vi "FPGA VI_8 Channels_High Speed.vi"() -> ()   [LabVIEW 2015]
uses:
  FPGA/Injection Capture IP/Types/Injection.Timing.ctl
  FPGA/Injection Capture IP/Types/Injection.Core.Settings.ctl
  FPGA/Injection Capture IP/Types/Injection.Global.Settings.ctl
  <vilib>/rvi/eio/common/nirviEmuClasses.ctl
  FPGA/Injection Capture IP/Types/Injection.Mux.State.ctl
  <vilib>/Platform/TimedLoop/XDataNode/timing_clust.ctl
  <vilib>/Platform/TimedLoop/XDataNode/nitl_modes.ctl
  <vilib>/Platform/TimedLoop/XDataNode/wakeup.ctl
  FPGA/Injection Capture IP/Types/Injection.Core.Internal.Settings.ctl
  <vilib>/rvi/eio/common/nirviEmuTemplateMethod_errors.vi
  <vilib>/rvi/Emulation/niFpgaGetClockAttributes.vi
  <vilib>/rvi/Emulation/niFpgaSctlEmulationGetInTimedLoop.vi
  <vilib>/rvi/Emulation/niFpgaEmulationReportErrorSimple.vi
  <vilib>/rvi/Emulation/niFpgaCriticalErrorInLSC.vi
  <vilib>/rvi/eio/common/nirviEmuTemplateMethod_noerrors.vi
  <vilib>/rvi/DataTransferAndStorage/Container/Common/niFpgaContainerExecOnDevCompGetState.vi
  <vilib>/rvi/Emulation/niFpgaEmulationIsFPGAContextNoSignature.vi
  <vilib>/rvi/errors/niFpgaSetErrorForExecOnDevCompSimple.vi
  <vilib>/rvi/eio/common/nirviEmuReportErrorAndStop.vi
  <vilib>/rvi/DataTransferAndStorage/Container/Common/niFpgaContainerGetUniqueNameForEmu.vi
  <vilib>/rvi/FIFO/Fifo_Resource/nirvififoEmulationSetSize.vi
  <vilib>/rvi/FIFO/Fifo_Resource/nirviFifoEmulationQueueMgr.vi
  <instcachedir>/0/nirviFifoEmulationQueueMgr_E5CAEC123FF24DC58D834DCA3CDAA9B5.lvgen/nirviFifoEmulationQueueMgr_E5CAEC123FF24DC58D834DCA3CDAA9B5_010.vi
  <vilib>/rvi/FIFO/Fifo_Resource/nirvififoEmulationDetermineInputValidOut.vi
  <vilib>/rvi/FIFO/Fifo_Resource/nirvififoEmulationCreateLock.vi
  <vilib>/rvi/Emulation/niFpgaProcessEmulError.vi
  <vilib>/rvi/FIFO/Fifo_Resource/nirvififoEmulationObtainLock.vi
  <vilib>/rvi/FIFO/Fifo_Resource/nirvififoEmulationReleaseLock.vi
  <vilib>/rvi/occurrence/nirviWaitOnOccurrenceBase.vi
  <vilib>/rvi/errors/nirviReportUnexpectedCaseInternalError.vi
  <vilib>/rvi/errors/nirviReportUnexpectedCaseInternalError (U32).vi
  <vilib>/Utility/error.llb/Clear Errors.vi
  <vilib>/rvi/interface/RandomDataEmulation/niFpgaRandomDataHandleErrors.vi
  <instcachedir>/0/nirviFifoEmulationQueueMgr_E5CAEC123FF24DC58D834DCA3CDAA9B5.lvgen/nirviFifoEmulationQueueMgr_E5CAEC123FF24DC58D834DCA3CDAA9B5_008.vi
  <vilib>/eio/EIOGrowableMethodNode/genericMethod/EIOGrowableMethodNode.xnode
  <vilib>/rvi/eio/nirviEIOMethodImplementation/nirviEIOMethodImplementation.xnode
  <vilib>/rvi/eio/nirviErrorMerge/nirviErrorMerge.xnode
  <vilib>/Platform/TimedLoop/XDataNode/XDataNode.xnode
  <vilib>/rvi/DataTransferAndStorage/Container/XNode/niFpgaContainer.xnode
  <vilib>/rvi/FIFO/Fifo_Resource/niFpgaFifoEmulationRefIn.vi
  <vilib>/rvi/interface/RandomDataEmulation/nirviRandomDataFpgaReadWriteTemplate.vi
  <vilib>/Platform/TimedLoop/XDataNode/XDNodeRunTimeDep.lvlib
panel:
  in  "Settings.DMA":cluster{"# of Injectors":u8}={"# of Injectors"=6}
  out "Host DMA Out?":bool
  out "Intermediate Time Out?":bool
  out "Sample Clock Ticks":u32
  out "Module Error":bool
  out "Module Initialization Error Code":i32
  out "IO Node Timeout":bool
  in  "Settings.Index6.Injectors.Injector6":T1
  in  "Settings.Index7.Injectors.Injector7":T1
  out "Intermediate FIFO Write Timeout":bool
  in  "Settings.Global.Injectors":T2={"Enable?"=FALSE, "Initial Voltage Threshold"=12.0, "Event Dwell Limit"=2000, "Voltage Gain"=1.0, "Current Gain"=1.0, "Filter Samples"=5, "Pretrigger Samples"=5}
  in  "Settings.Index0.Injectors.Injector0":T1
  in  "Settings.Index1.Injectors.Injector1":T1
  in  "Settings.Index2.Injectors.Injector2":T1
  in  "Settings.Index3.Injectors.Injector3":T1
  in  "Settings.Index4.Injectors.Injector4":T1
  in  "Settings.Index5.Injectors.Injector5":T1
  in  "Settings.Timing":T3={"Injection Sample Period (Ticks)"=80}
  out "Acqusition Loop Ticks":u32
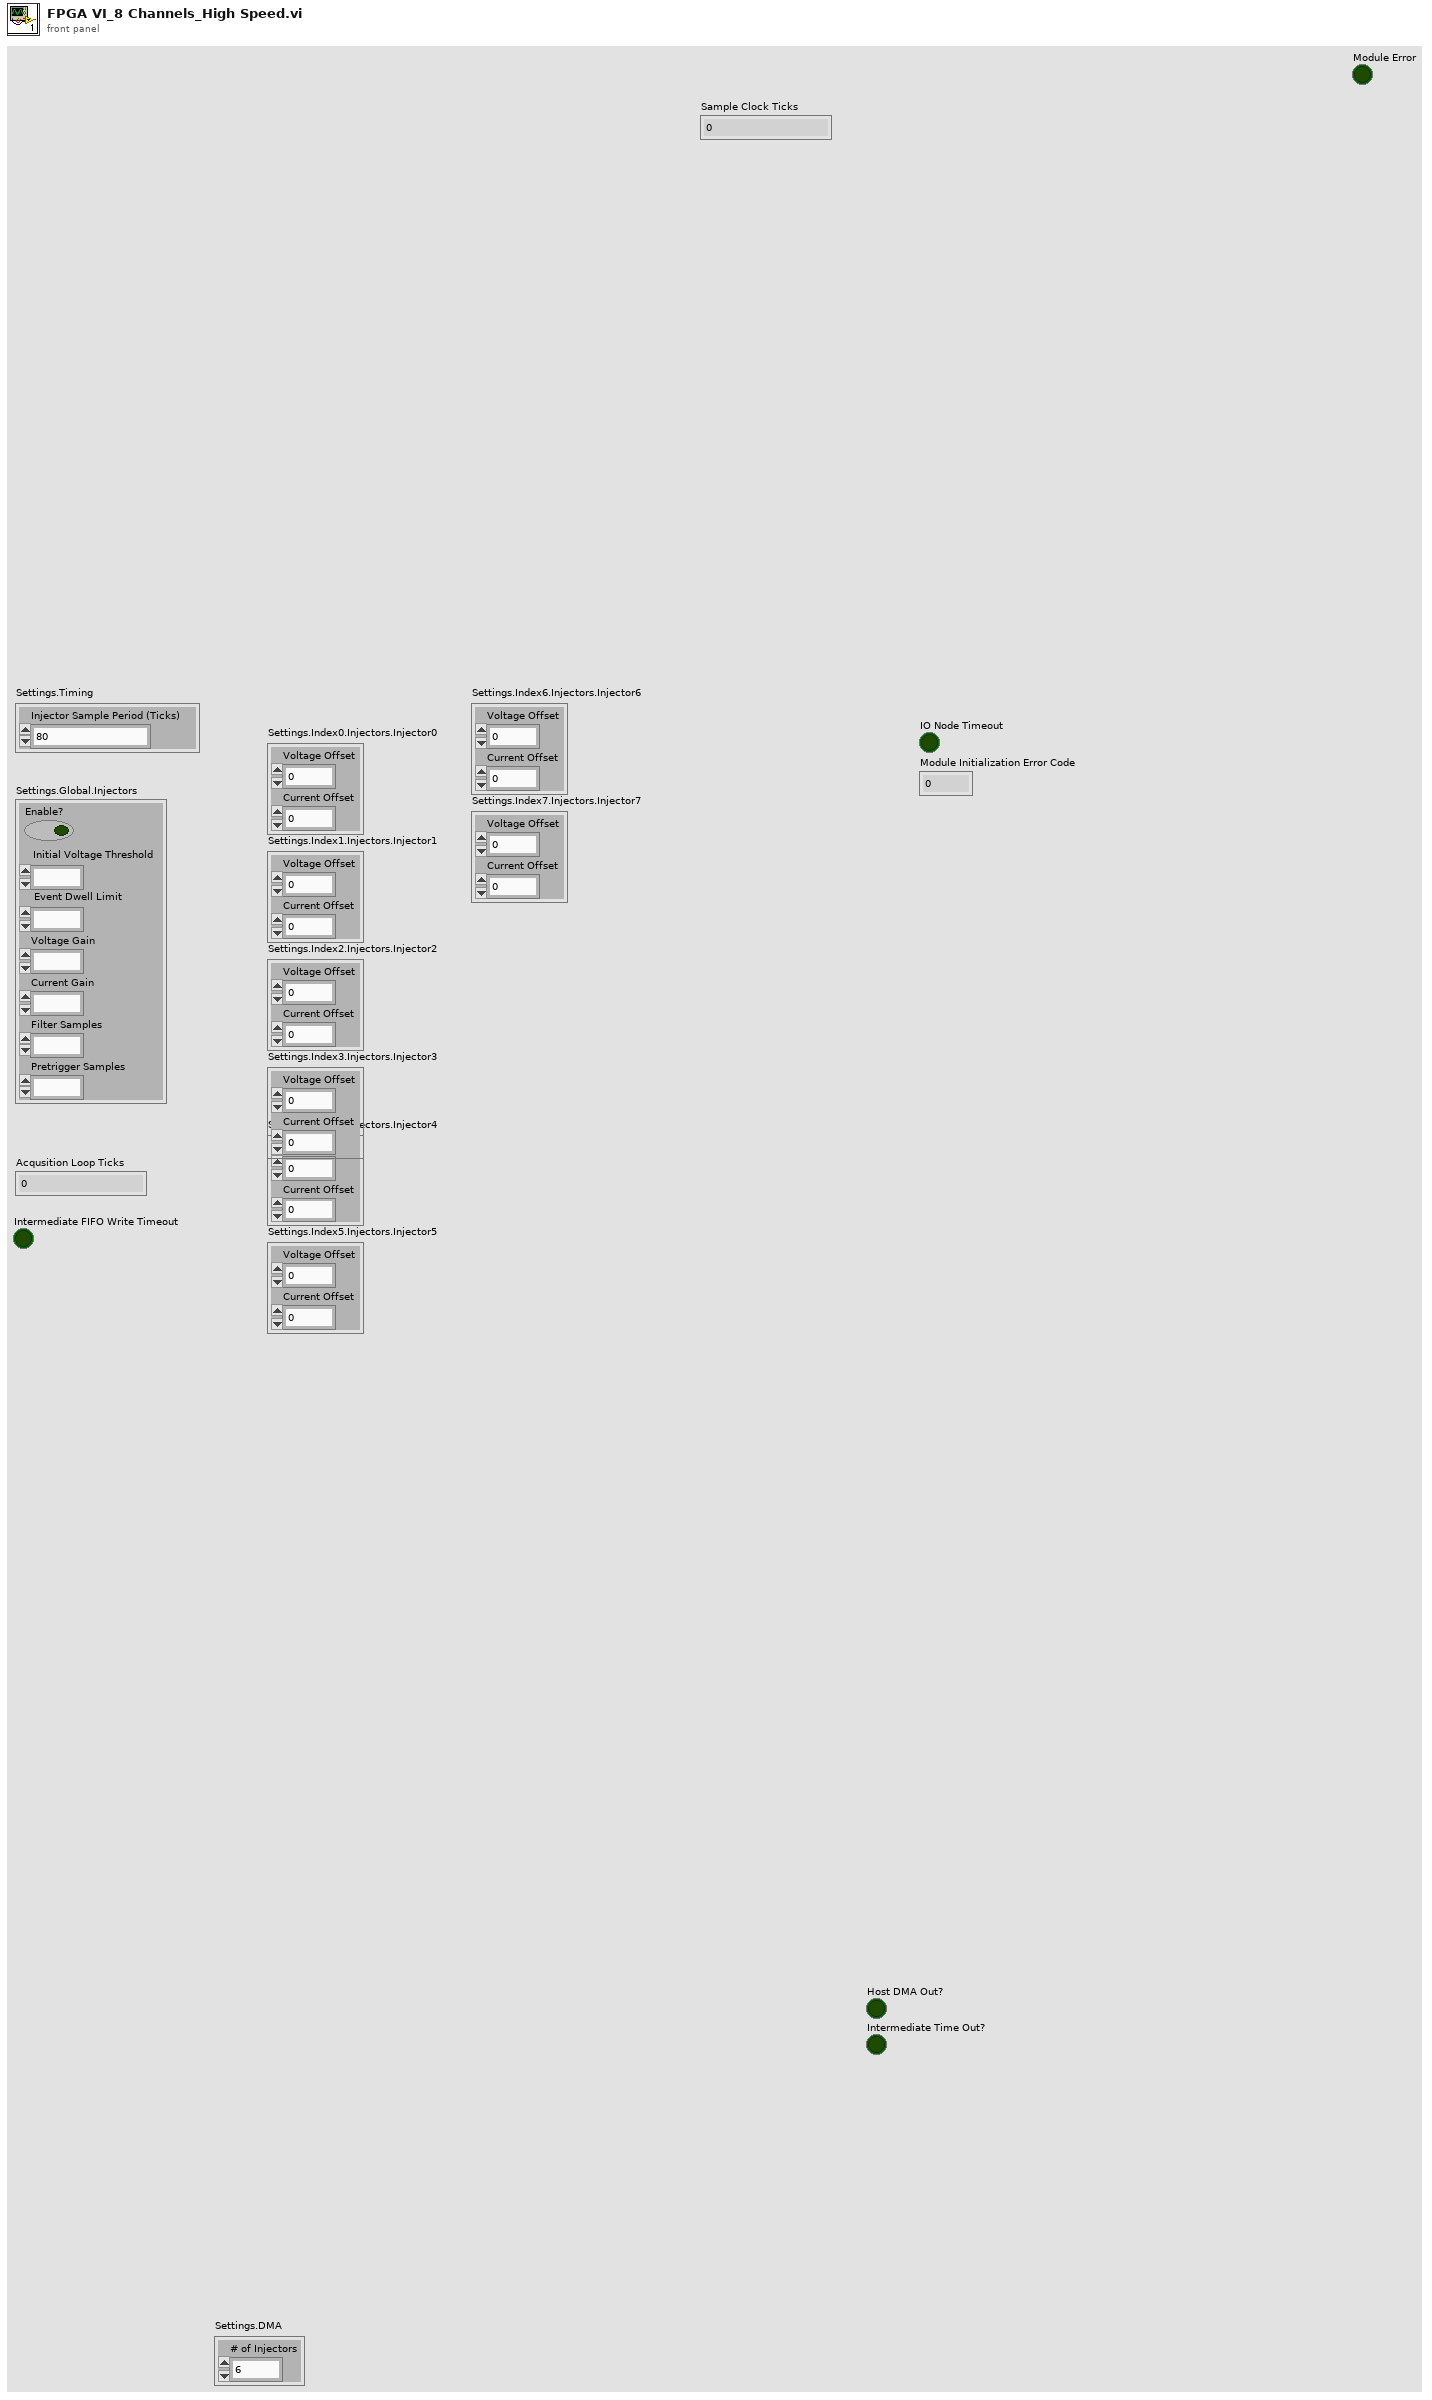
[diagram p1: front panel]
types:
  T1 = typedef "Injection.Core.Settings.ctl" = cluster{"Voltage Offset":fxp<+/-,32,8>, "Current Offset":fxp<+/-,32,8>}
  T2 = typedef "Injection.Global.Settings.ctl" = cluster{"Enable?":bool, "Initial Voltage Threshold":fxp<+/-,32,8>, "Event Dwell Limit":u16, "Voltage Gain":fxp<+/-,32,8>, "Current Gain":fxp<+/-,32,8>, "Filter Samples":u8, "Pretrigger Samples":u8}
  T3 = typedef "Injection.Timing.ctl" = cluster{"Injection Sample Period (Ticks)":u32}
  T4 = typedef "nirviEmuClasses.ctl" = enum16{"IO Read", "IO Write", "Method", "Property Read", "Property Write"}
  T5 = cluster{"Data.Samples":u32, "Injection.Period":u32, "Injector.Index":u8, "Iteration":u32}
  T6 = typedef "Injection.Mux.State.ctl" = enum8{"Wait on Transfer", "Transfer Injector Index", "Transfer # of Samples", "Transfer Injection Period", "Transfer Data Samples"}
  T7 = typedef "XDNodeRunTimeDep.lvlib/timing_clust.ctl" = cluster{"Expected End [f-1]":u64, "Actual End [f-1]":u64, "Finished Late? [f-1]":bool, "Expected End [i-1]":u64, "Actual End [i-1]":u64, "Finished Late? [i-1]":bool, "Expected Start [i]":u64, "Actual Start [i]":u64, "Expected Start [f]":u64, "Actual Start [f]":u64, "Source Name":string, "Structure Name":string, "Period":i64, "Deadline":i64, "Offset":i64, "Start":i64, "Priority":i32, "Timeout":i32, "Mode":T8, "Wakeup Reason":T9, "Error":errorcluster, "Source Type":string, "Secondary Source Type":string, "Global End Time":u64, "Global Start Time":u64, "Frame Duration":u64, "Iteration Duration":u64, "Assigned CPU":i32, "I/O Scan Engine Mode":u32}
  T8 = typedef "XDNodeRunTimeDep.lvlib/nitl_modes.ctl" = enum32{"No Change", "Process missed periods, maintain original phase", "Discard missed periods, maintain original phase", "Process missed periods, ignore original phase", "Discard missed periods, ignore original phase"}
  T9 = typedef "XDNodeRunTimeDep.lvlib/wakeup.ctl" = enum32{"Normal", "Aborted", "Asynchronous wakeup", "Timing source error", "Timed loop error", "Timeout"}
  T10 = typedef "Injection.Core.Internal.Settings.ctl" = cluster{"Data Buffer FIFO":refnum<k21>, "Capture Complete Trigger FIFO":refnum<k21>}
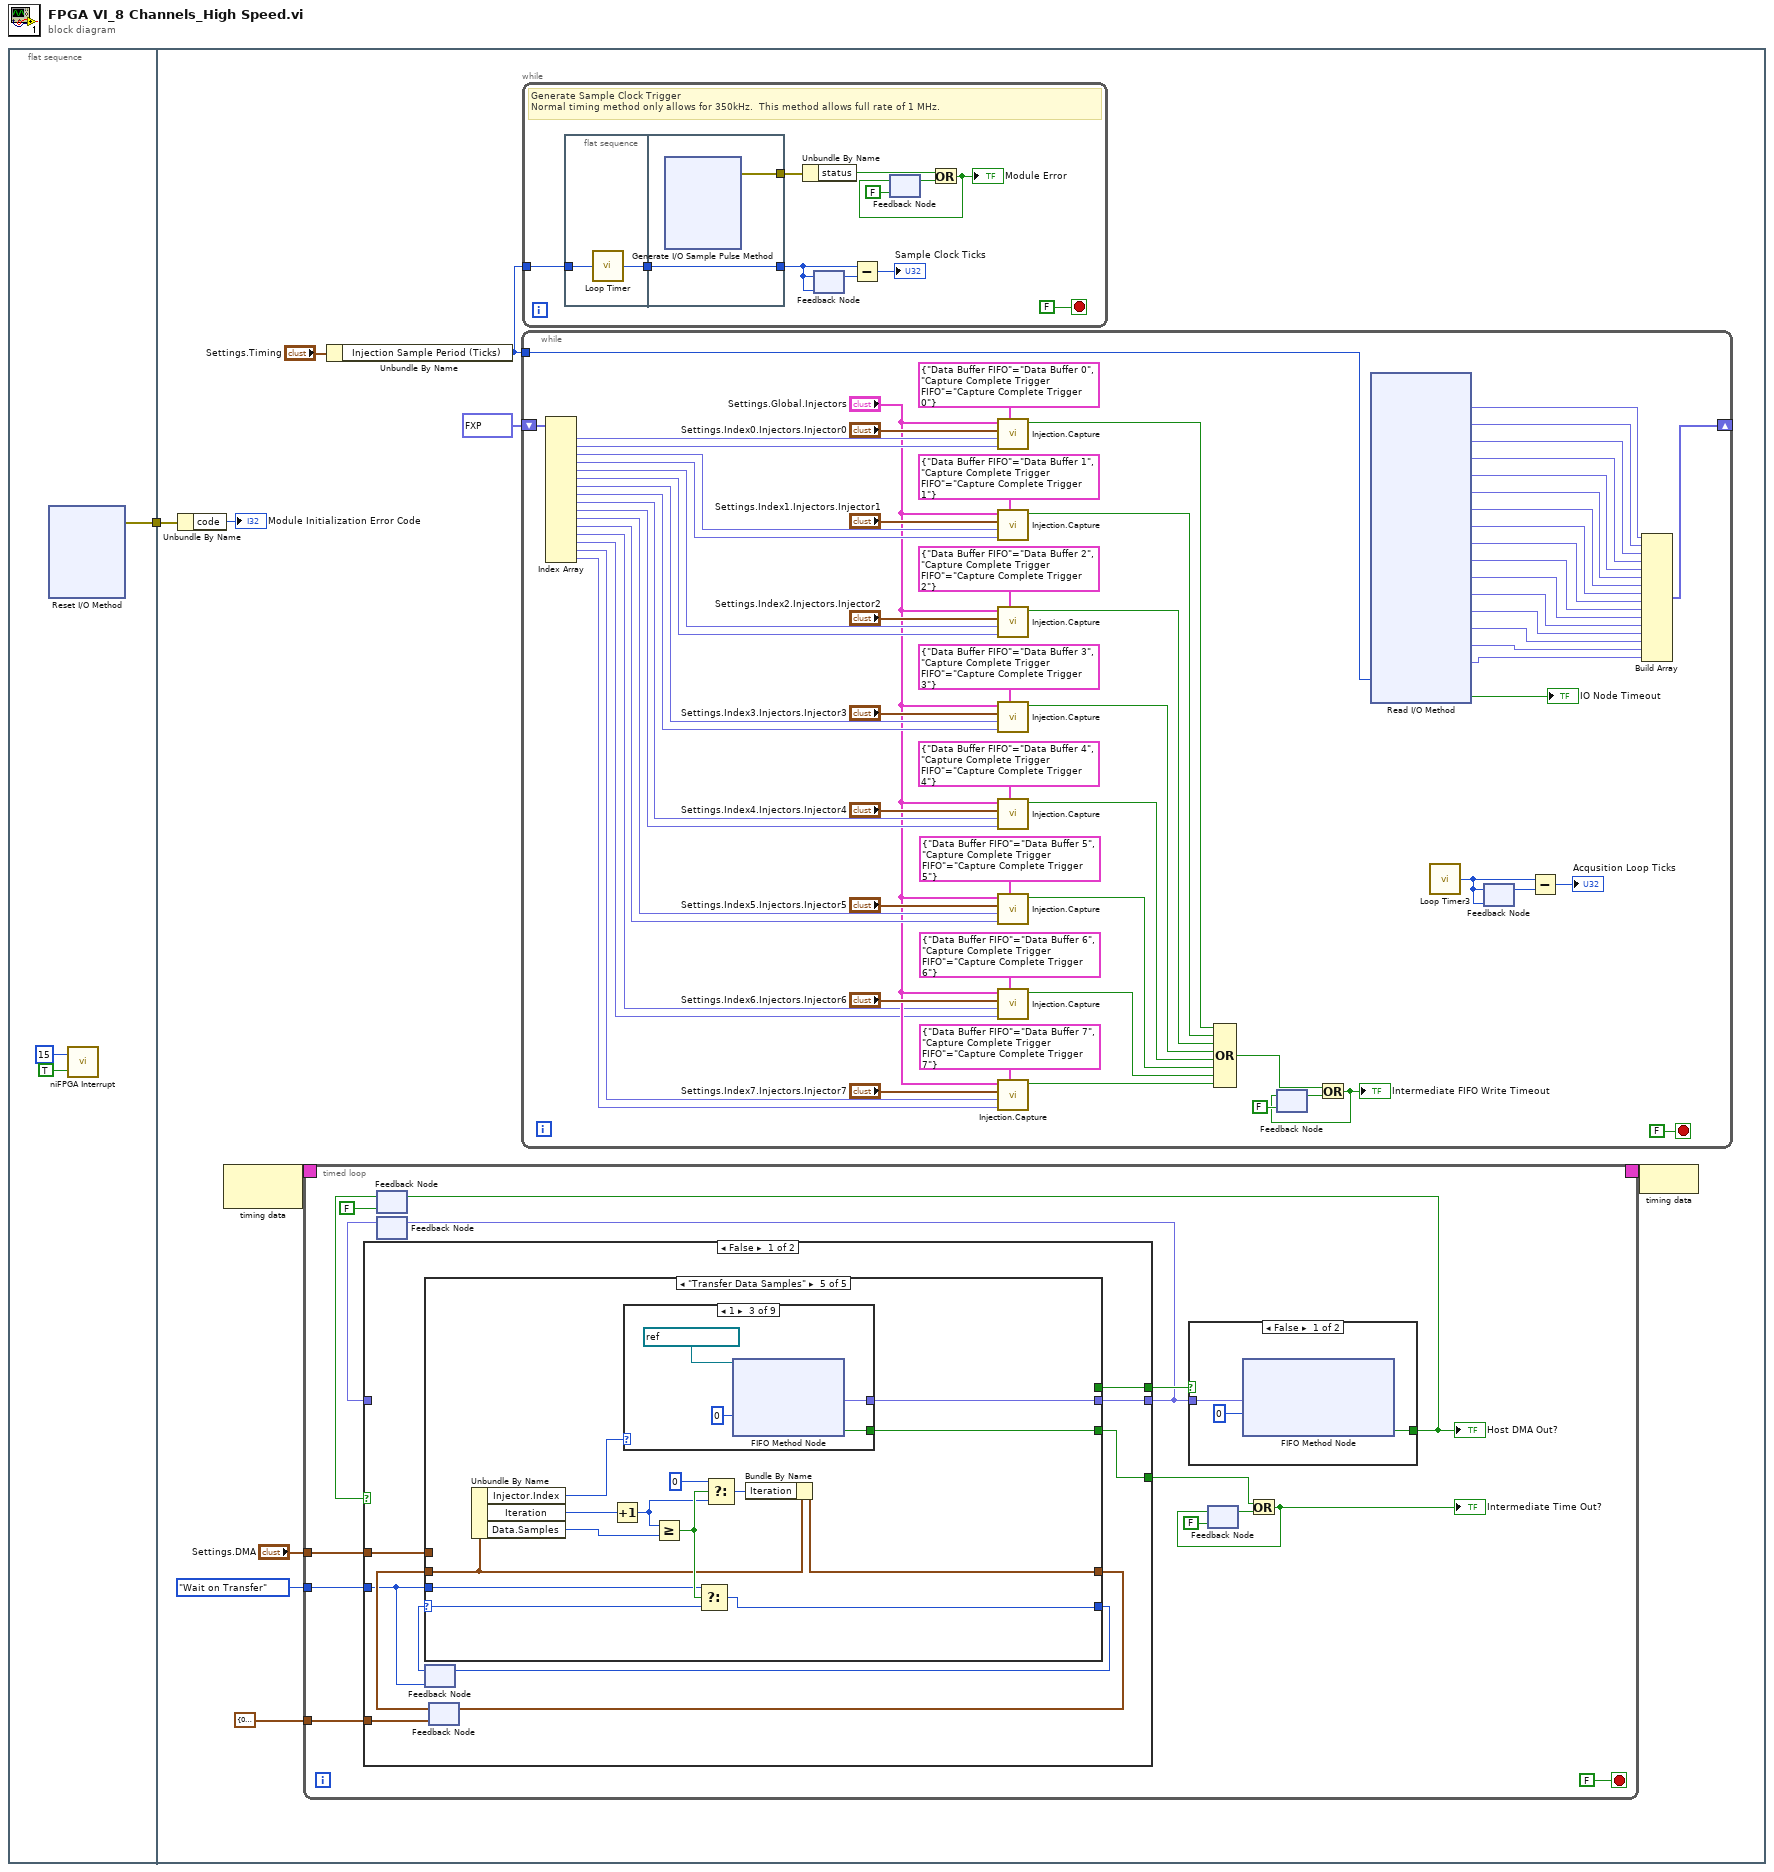
[diagram p0: block diagram]
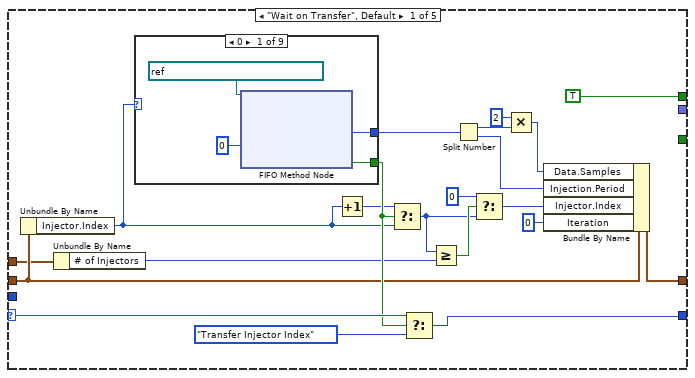
[diagram p2: hidden frame]
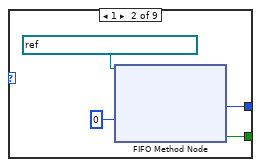
[diagram p3: hidden frame]
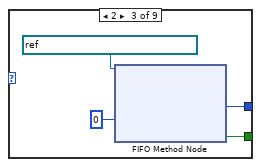
[diagram p4: hidden frame]
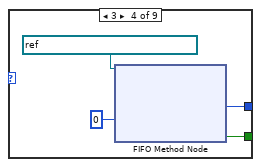
[diagram p5: hidden frame]
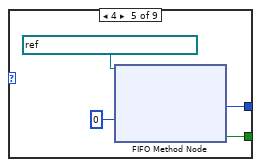
[diagram p6: hidden frame]
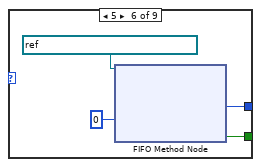
[diagram p7: hidden frame]
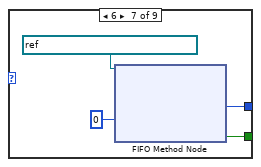
[diagram p8: hidden frame]
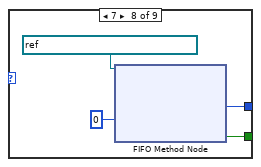
[diagram p9: hidden frame]
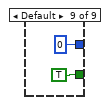
[diagram p10: hidden frame]
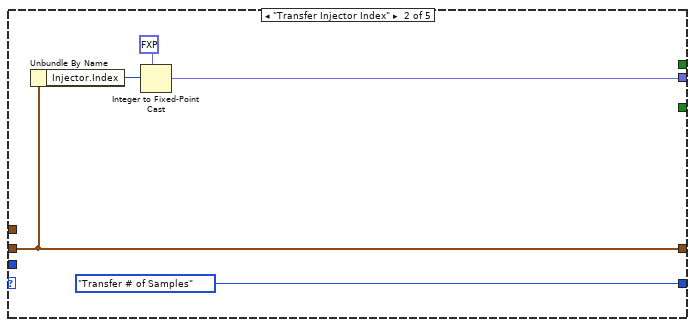
[diagram p11: hidden frame]
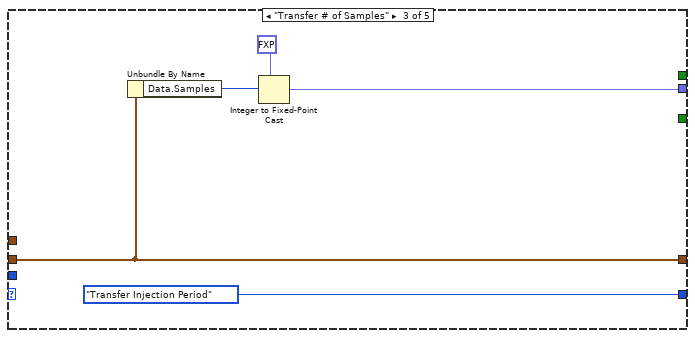
[diagram p12: hidden frame]
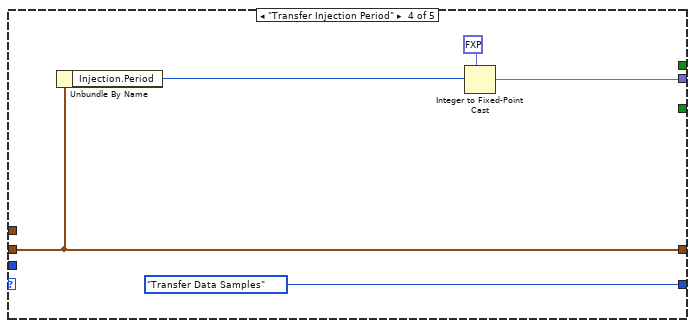
[diagram p13: hidden frame]
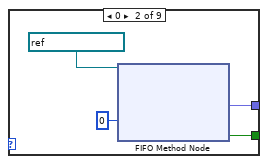
[diagram p15: hidden frame]
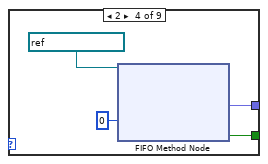
[diagram p16: hidden frame]
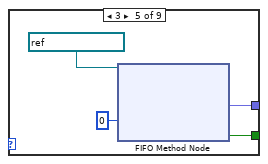
[diagram p17: hidden frame]
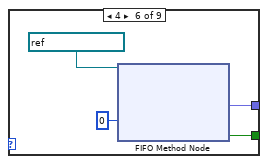
[diagram p18: hidden frame]
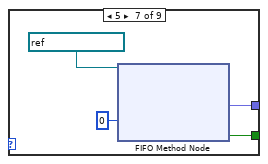
[diagram p19: hidden frame]
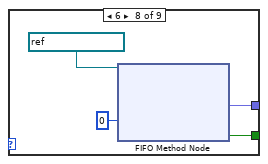
[diagram p20: hidden frame]
diagram:
  n1 = flat-sequence {
    tunnel: [w2] -> w1
    tunnel: w1 -> [w86]
    frame #0 {
      n2 = xnode "Reset I/O Method"() -> ("error out"=w2:errorcluster)  [unwired: 5 in, 4 out]
      n3 = call <vilib>:"niFPGA Interrupt.vi"("Wait Until Cleared (F)"=TRUE, "IRQ Number (0)"=u8 15) -> ()  [unwired: 1 in]
    }
    frame #1 {
      n4 = Unbundle By Name(w86) -> ("code"=→"Module Initialization Error Code":i32)
      n5 = node-c288() -> (w83:T7)  [unwired: 1 in]
      n6 = timed-loop {
        timing: w83 -> [_]
        timing-out: [_] -> w82
        tunnel: "Settings.DMA" -> [w92]
        tunnel: Injection.Mux.State."Wait on Transfer" -> [w91]
        tunnel: T5 {"Data.Samples"=0, "Injection.Period"=0, "Injector.Index"=0, "Iteration"=0} ("Local.Data") -> [w90]
        stop <- FALSE stop-if-true
        n7 = feedback #1(FALSE ("Timed Out?")) -> (w100:bool)
        n8 = feedback #2() -> (w97:fxp<+/-,32,8>)  [unwired: 1 in]
        n9 = case shown="False" w100 {
          tunnel: [w112 w230] -> w98
          tunnel: [w111 w229] -> w102
          tunnel: w91 -> [w105 _]
          tunnel: [w110 w229] -> w93
          tunnel: w92 -> [w109 _]
          tunnel: w90 -> [w106 _]
          tunnel: w97 -> [_ w230]
          frame False {
            n10 = feedback #3(w105) -> (w104:T6)
            n11 = feedback #4(w106) -> (w107:T5)
            n12 = case shown="\"Transfer Data Samples\"" w104 {
              selector: w104 -> [w133 _ _ _ w190]
              tunnel: w107 -> [w124 w171 w175 w179 w188]
              tunnel: [w132 w171 w175 w179 w187] -> w108
              tunnel: [w131 Injection.Mux.State."Transfer # of Samples" Injection.Mux.State."Transfer Injection Period" Injection.Mux.State."Transfer Data Samples" w189] -> w103
              tunnel: [_ w170 w174 w181 w186] -> w112
              tunnel: [TRUE _ _ _ _] -> w111
              tunnel: w105 -> [_ _ _ _ w183]
              tunnel: [_ _ _ _ w185] -> w110
              tunnel: w109 -> [w121 _ _ _ _]
              frame "Wait on Transfer", Default {
                n13 = Unbundle By Name(w124) -> ("Injector.Index"=w123:u8)
                n14 = Unbundle By Name(w121) -> ("# of Injectors"=w120:u8)
                n15 = case shown="0" w123 {
                  tunnel: [w136 w140 w144 w148 w152 w156 w160 w164 u64 0 ("Element")] -> w119
                  tunnel: [w135 w139 w143 w147 w151 w155 w159 w163 TRUE ("Timed Out?")] -> w129
                  frame 0 {
                    n16 = xnode ("FIFO Method Node")("Timeout"=0, "FIFO In"=refnum<k21> "Capture Complete Trigger 0") -> ("Element"=w136:u64, "Timed Out?"=w135:bool)  [unwired: 1 out]
                  }
                  frame 1 {
                    n17 = xnode ("FIFO Method Node")("Timeout"=0, "FIFO In"=refnum<k21> "Capture Complete Trigger 1") -> ("Element"=w140:u64, "Timed Out?"=w139:bool)  [unwired: 1 out]
                  }
                  frame 2 {
                    n18 = xnode ("FIFO Method Node")("Timeout"=0, "FIFO In"=refnum<k21> "Capture Complete Trigger 2") -> ("Element"=w144:u64, "Timed Out?"=w143:bool)  [unwired: 1 out]
                  }
                  frame 3 {
                    n19 = xnode ("FIFO Method Node")("Timeout"=0, "FIFO In"=refnum<k21> "Capture Complete Trigger 3") -> ("Element"=w148:u64, "Timed Out?"=w147:bool)  [unwired: 1 out]
                  }
                  frame 4 {
                    n20 = xnode ("FIFO Method Node")("Timeout"=0, "FIFO In"=refnum<k21> "Capture Complete Trigger 4") -> ("Element"=w152:u64, "Timed Out?"=w151:bool)  [unwired: 1 out]
                  }
                  frame 5 {
                    n21 = xnode ("FIFO Method Node")("Timeout"=0, "FIFO In"=refnum<k21> "Capture Complete Trigger 5") -> ("Element"=w156:u64, "Timed Out?"=w155:bool)  [unwired: 1 out]
                  }
                  frame 6 {
                    n22 = xnode ("FIFO Method Node")("Timeout"=0, "FIFO In"=refnum<k21> "Capture Complete Trigger 6") -> ("Element"=w160:u64, "Timed Out?"=w159:bool)  [unwired: 1 out]
                  }
                  frame 7 {
                    n23 = xnode ("FIFO Method Node")("Timeout"=0, "FIFO In"=refnum<k21> "Capture Complete Trigger 7") -> ("Element"=w164:u64, "Timed Out?"=w163:bool)  [unwired: 1 out]
                  }
                  frame Default {
                  }
                }
                n24 = Increment(x=w123) -> (x+1=w128:u8)
                n25 = Select(t=w128, s=w129, f=w123) -> (s? t:f=w126:u8)
                n26 = Select(t=w133, s=w129, f=Injection.Mux.State."Transfer Injector Index") -> (s? t:f=w131:T6)
                n27 = Greater Or Equal?(x=w126, y=w120) -> (x >= y?=w127:bool)
                n28 = Split Number(x=w119) -> (hi(x)=w118:u32, lo(x)=w117:u32)
                n29 = Select(t=u8 0, s=w127, f=w126) -> (s? t:f=w122:u8)
                n30 = Multiply(x=u32 2, y=w118) -> (x*y=w115:u32)
                n31 = Bundle By Name(cluster=w124, "Data.Samples"=w115, "Injection.Period"=w117, "Injector.Index"=w122, "Iteration"=u32 0) -> (w132:T5)
              }
              frame "Transfer Injector Index" {
                n32 = Unbundle By Name(w171) -> ("Injector.Index"=w172:u8)
                n33 = Integer to Fixed-Point Cast(fixed-point type=fxp<+/-,32,8> 0.0, integer=w172) -> (fixed-point=w170:fxp<+/-,32,8>)
              }
              frame "Transfer # of Samples" {
                n34 = Unbundle By Name(w175) -> ("Data.Samples"=w176:u32)
                n35 = Integer to Fixed-Point Cast(fixed-point type=fxp<+/-,32,8> 0.0, integer=w176) -> (fixed-point=w174:fxp<+/-,32,8>)
              }
              frame "Transfer Injection Period" {
                n36 = Unbundle By Name(w179) -> ("Injection.Period"=w180:u32)
                n37 = Integer to Fixed-Point Cast(fixed-point type=fxp<+/-,32,8> 0.0, integer=w180) -> (fixed-point=w181:fxp<+/-,32,8>)
              }
              frame "Transfer Data Samples" {
                n38 = Unbundle By Name(w188) -> ("Injector.Index"=w196:u8, "Iteration"=w191:u32, "Data.Samples"=w184:u32)
                n39 = Increment(x=w191) -> (x+1=w193:u32)
                n40 = case shown="1" w196 {
                  tunnel: [_ w199 w203 w207 w211 w215 w219 w223 w227] -> w186
                  tunnel: [_ w198 w202 w206 w210 w214 w218 w222 w226] -> w185
                  frame Default {
                  }
                  frame 0 {
                    n41 = xnode ("FIFO Method Node")("Timeout"=0, "FIFO In"=refnum<k21> "Data Buffer 0" ("Voltage FIFO")) -> ("Element"=w199:fxp<+/-,32,8>, "Timed Out?"=w198:bool)  [unwired: 1 out]
                  }
                  frame 1 {
                    n42 = xnode ("FIFO Method Node")("Timeout"=0, "FIFO In"=refnum<k21> "Data Buffer 1" ("Voltage FIFO")) -> ("Element"=w203:fxp<+/-,32,8>, "Timed Out?"=w202:bool)  [unwired: 1 out]
                  }
                  frame 2 {
                    n43 = xnode ("FIFO Method Node")("Timeout"=0, "FIFO In"=refnum<k21> "Data Buffer 2" ("Voltage FIFO")) -> ("Element"=w207:fxp<+/-,32,8>, "Timed Out?"=w206:bool)  [unwired: 1 out]
                  }
                  frame 3 {
                    n44 = xnode ("FIFO Method Node")("Timeout"=0, "FIFO In"=refnum<k21> "Data Buffer 3" ("Voltage FIFO")) -> ("Element"=w211:fxp<+/-,32,8>, "Timed Out?"=w210:bool)  [unwired: 1 out]
                  }
                  frame 4 {
                    n45 = xnode ("FIFO Method Node")("Timeout"=0, "FIFO In"=refnum<k21> "Data Buffer 4" ("Voltage FIFO")) -> ("Element"=w215:fxp<+/-,32,8>, "Timed Out?"=w214:bool)  [unwired: 1 out]
                  }
                  frame 5 {
                    n46 = xnode ("FIFO Method Node")("Timeout"=0, "FIFO In"=refnum<k21> "Data Buffer 5" ("Voltage FIFO")) -> ("Element"=w219:fxp<+/-,32,8>, "Timed Out?"=w218:bool)  [unwired: 1 out]
                  }
                  frame 6 {
                    n47 = xnode ("FIFO Method Node")("Timeout"=0, "FIFO In"=refnum<k21> "Data Buffer 6" ("Voltage FIFO")) -> ("Element"=w223:fxp<+/-,32,8>, "Timed Out?"=w222:bool)  [unwired: 1 out]
                  }
                  frame 7 {
                    n48 = xnode ("FIFO Method Node")("Timeout"=0, "FIFO In"=refnum<k21> "Data Buffer 7" ("Voltage FIFO")) -> ("Element"=w227:fxp<+/-,32,8>, "Timed Out?"=w226:bool)  [unwired: 1 out]
                  }
                }
                n49 = Greater Or Equal?(x=w193, y=w184) -> (x >= y?=w195:bool)
                n50 = Select(t=w183, s=w195, f=w190) -> (s? t:f=w189:T6)
                n51 = Select(t=u32 0, s=w195, f=w193) -> (s? t:f=w192:u32)
                n52 = Bundle By Name(cluster=w188, "Iteration"=w192) -> (w187:T5)
              }
            }
            n53 = feedback-in #3(w103) -> ()
            n54 = feedback-in #4(w108) -> ()
          }
          frame True {
            w229 = FALSE
          }
        }
        n55 = feedback-in #2(w98) -> ()
        n56 = case shown="False" w102 {
          tunnel: w98 -> [w232 _]
          tunnel: [w231 FALSE ("Timed Out?")] -> w101
          frame False {
            n57 = xnode ("FIFO Method Node")("Element"=w232, "Timeout"=0) -> ("Timed Out?"=w231:bool)  [unwired: 1 in, 1 out]
          }
          frame True {
          }
        }
        "Host DMA Out?" <- w101
        n58 = feedback-in #1(w101) -> ()
        n59 = feedback #5(FALSE ("Timed Out?")) -> (w95:bool)
        n60 = Or(x=w93, y=w95) -> (x .or. y?=w94:bool)
        "Intermediate Time Out?" <- w94
        n61 = feedback-in #5(w94) -> ()
      }
      n62 = Unbundle By Name("Settings.Timing") -> ("Injection Sample Period (Ticks)"=w84:u32)
      n63 = while {
        shift-right: [w268] -> _
        shift-left: fxp<+/-,24,5>[] [0.0, 0.0, 0.0, 0.0, 0.0, 0.0, 0.0, 0.0, 0.0, 0.0, 0.0, 0.0, 0.0, 0.0, 0.0, 0.0] -> [w288]
        tunnel: w84 -> [w239]
        stop <- FALSE stop-if-true
        n64 = Index Array(array=w288) -> (element #1=w299:fxp<+/-,24,5>, element #2=w300:fxp<+/-,24,5>, element #3=w297:fxp<+/-,24,5>, element #4=w298:fxp<+/-,24,5>, element #5=w295:fxp<+/-,24,5>, element #6=w296:fxp<+/-,24,5>, element #7=w293:fxp<+/-,24,5>, element #8=w294:fxp<+/-,24,5>, element #9=w291:fxp<+/-,24,5>, element #10=w292:fxp<+/-,24,5>, element #11=w289:fxp<+/-,24,5>, element #12=w290:fxp<+/-,24,5>, element #13=w260:fxp<+/-,24,5>, element #14=w259:fxp<+/-,24,5>, element #15=w258:fxp<+/-,24,5>, element #16=w257:fxp<+/-,24,5>)  [unwired: 16 in]
        n65 = call "Injection.Capture.vi"("FIFOs"=T10 {"Data Buffer FIFO"="Data Buffer 0", "Capture Complete Trigger FIFO"="Capture Complete Trigger 0"} ("InjectorCore.Settings"), "Current (PreScaled)"=w300, "Voltage (PreScaled)"=w299, "Settings.Index<#>.<Group>.<UserName>"="Settings.Index0.Injectors.Injector0", "Settings.Global.<Group>"="Settings.Global.Injectors") -> ("Intermediate FIFO Timeout?"=w307:bool)  [unwired: 4 in, 2 out]
        n66 = call "Injection.Capture.vi"("FIFOs"=T10 {"Data Buffer FIFO"="Data Buffer 1", "Capture Complete Trigger FIFO"="Capture Complete Trigger 1"} ("InjectorCore.Settings"), "Current (PreScaled)"=w298, "Voltage (PreScaled)"=w297, "Settings.Index<#>.<Group>.<UserName>"="Settings.Index1.Injectors.Injector1", "Settings.Global.<Group>"="Settings.Global.Injectors") -> ("Intermediate FIFO Timeout?"=w306:bool)  [unwired: 4 in, 2 out]
        n67 = call "Injection.Capture.vi"("FIFOs"=T10 {"Data Buffer FIFO"="Data Buffer 2", "Capture Complete Trigger FIFO"="Capture Complete Trigger 2"} ("InjectorCore.Settings"), "Current (PreScaled)"=w296, "Voltage (PreScaled)"=w295, "Settings.Index<#>.<Group>.<UserName>"="Settings.Index2.Injectors.Injector2", "Settings.Global.<Group>"="Settings.Global.Injectors") -> ("Intermediate FIFO Timeout?"=w305:bool)  [unwired: 4 in, 2 out]
        n68 = call "Injection.Capture.vi"("FIFOs"=T10 {"Data Buffer FIFO"="Data Buffer 3", "Capture Complete Trigger FIFO"="Capture Complete Trigger 3"} ("InjectorCore.Settings"), "Current (PreScaled)"=w294, "Voltage (PreScaled)"=w293, "Settings.Index<#>.<Group>.<UserName>"="Settings.Index3.Injectors.Injector3", "Settings.Global.<Group>"="Settings.Global.Injectors") -> ("Intermediate FIFO Timeout?"=w304:bool)  [unwired: 4 in, 2 out]
        n69 = call "Injection.Capture.vi"("FIFOs"=T10 {"Data Buffer FIFO"="Data Buffer 4", "Capture Complete Trigger FIFO"="Capture Complete Trigger 4"} ("InjectorCore.Settings"), "Current (PreScaled)"=w292, "Voltage (PreScaled)"=w291, "Settings.Index<#>.<Group>.<UserName>"="Settings.Index4.Injectors.Injector4", "Settings.Global.<Group>"="Settings.Global.Injectors") -> ("Intermediate FIFO Timeout?"=w303:bool)  [unwired: 4 in, 2 out]
        n70 = call "Injection.Capture.vi"("FIFOs"=T10 {"Data Buffer FIFO"="Data Buffer 5", "Capture Complete Trigger FIFO"="Capture Complete Trigger 5"} ("InjectorCore.Settings"), "Current (PreScaled)"=w290, "Voltage (PreScaled)"=w289, "Settings.Index<#>.<Group>.<UserName>"="Settings.Index5.Injectors.Injector5", "Settings.Global.<Group>"="Settings.Global.Injectors") -> ("Intermediate FIFO Timeout?"=w302:bool)  [unwired: 4 in, 2 out]
        n71 = call "Injection.Capture.vi"("FIFOs"=T10 {"Data Buffer FIFO"="Data Buffer 6", "Capture Complete Trigger FIFO"="Capture Complete Trigger 6"} ("InjectorCore.Settings"), "Current (PreScaled)"=w259, "Voltage (PreScaled)"=w260, "Settings.Index<#>.<Group>.<UserName>"="Settings.Index6.Injectors.Injector6", "Settings.Global.<Group>"="Settings.Global.Injectors") -> ("Intermediate FIFO Timeout?"=w262:bool)  [unwired: 4 in, 2 out]
        n72 = call "Injection.Capture.vi"("FIFOs"=T10 {"Data Buffer FIFO"="Data Buffer 7", "Capture Complete Trigger FIFO"="Capture Complete Trigger 7"} ("InjectorCore.Settings"), "Current (PreScaled)"=w257, "Voltage (PreScaled)"=w258, "Settings.Index<#>.<Group>.<UserName>"="Settings.Index7.Injectors.Injector7", "Settings.Global.<Group>"="Settings.Global.Injectors") -> ("Intermediate FIFO Timeout?"=w261:bool)  [unwired: 4 in, 2 out]
        n73 = Compound Arithmetic op=OR(w307, w306, w305, w304, w303, w302, w262, w261) -> (w278:bool)
        n74 = feedback #6(FALSE ("Timed Out?")) -> (w279:bool)
        n75 = Or(x=w278, y=w279) -> (x .or. y?=w277:bool)
        "Intermediate FIFO Write Timeout" <- w277
        n76 = feedback-in #6(w277) -> ()
        n77 = xnode "Read I/O Method"("Timeout"=w239) -> ("Mod1/AI0"=w256:fxp<+/-,24,5>, "Mod1/AI1"=w255:fxp<+/-,24,5>, "Mod1/AI2"=w254:fxp<+/-,24,5>, "Mod1/AI3"=w253:fxp<+/-,24,5>, "Mod2/AI0"=w252:fxp<+/-,24,5>, "Mod2/AI1"=w251:fxp<+/-,24,5>, "Mod2/AI2"=w250:fxp<+/-,24,5>, "Mod2/AI3"=w249:fxp<+/-,24,5>, "Mod3/AI0"=w248:fxp<+/-,24,5>, "Mod3/AI1"=w247:fxp<+/-,24,5>, "Mod3/AI2"=w246:fxp<+/-,24,5>, "Mod3/AI3"=w245:fxp<+/-,24,5>, "Mod4/AI0"=w244:fxp<+/-,24,5>, "Mod4/AI1"=w243:fxp<+/-,24,5>, "Mod4/AI2"=w242:fxp<+/-,24,5>, "Mod4/AI3"=w241:fxp<+/-,24,5>, "Timed Out"=→"IO Node Timeout":bool)  [unwired: 17 in, 17 out]
        n78 = call "Loop Timer3"() -> ("Tick Count(Ticks)"=w274:u32)  [unwired: 1 in]
        n79 = feedback #7(w274) -> (w276:u32)
        n80 = feedback-in #7(w274) -> ()
        n81 = Subtract(x=w274, y=w276) -> (x-y=→"Acqusition Loop Ticks":u32)
        n82 = Build Array(w256, w255, w254, w253, w252, w251, w250, w249, w248, w247, w246, w245, w244, w243, w242, w241) -> (w268:fxp<+/-,24,5>[])
      }
      n83 = while {
        tunnel: w84 -> [w831]
        stop <- FALSE stop-if-true
        # "Generate Sample Clock Trigger\nNormal timing method only allows for 350kHz.  This method allows full rate of 1 MHz."
        n84 = flat-sequence {
          tunnel: w831 -> [w834]
          tunnel: [w833] -> w822
          tunnel: [w836] -> w832
          tunnel: [w835] -> w823
          tunnel: w822 -> [w835]
          frame #0 {
            n85 = call "Loop Timer"("Count(Ticks)"=w834) -> ("Tick Count(Ticks)"=w833:u32)
          }
          frame #1 {
            n86 = xnode "Generate I/O Sample Pulse Method"() -> ("error out"=w836:errorcluster)  [unwired: 5 in, 4 out]
          }
        }
        n87 = Unbundle By Name(w832) -> ("status"=w824:bool)
        n88 = feedback #8(w823) -> (w829:u32)
        n89 = feedback-in #8(w823) -> ()
        n90 = Subtract(x=w823, y=w829) -> (x-y=→"Sample Clock Ticks":u32)
        n91 = feedback #9(FALSE ("Timed Out?")) -> (w826:bool)
        n92 = Or(x=w824, y=w826) -> (x .or. y?=w825:bool)
        "Module Error" <- w825
        n93 = feedback-in #9(w825) -> ()
      }
      n94 = node-c288(w82) -> ()
    }
  }
